vi "shift Scan Pattern.vi"(4 "error in (no error)":errorcluster, 5 "Shift Y":dbl, 6 "Shift X":dbl, 7 "Scan Pattern in":refnum<class "Scan Pattern.lvclass">) -> (0 "error out":errorcluster, 3 "Scan Pattern out":refnum<class "Scan Pattern.lvclass">)   [LabVIEW 2018]
uses:
  SpectralRadar/LabVIEW/2012/user.lib/SpectralRadar.llb/Scan Pattern.lvclass
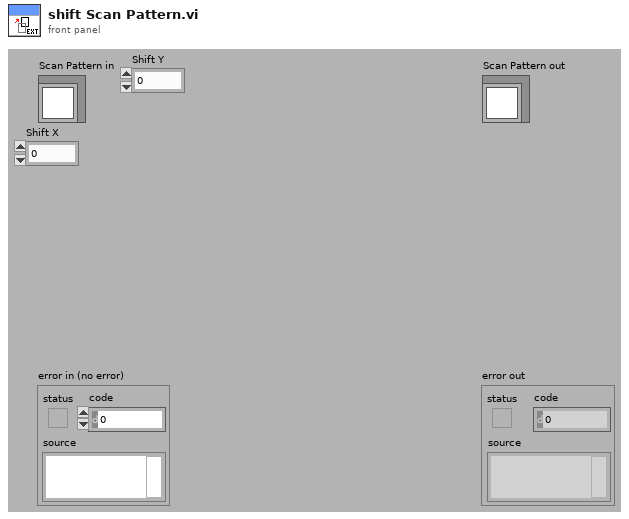
[diagram p1: front panel]
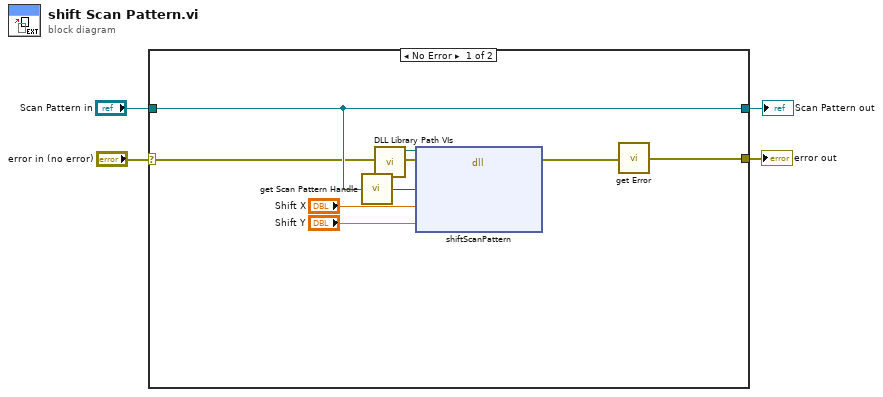
[diagram p0: block diagram]
diagram:
  n1 = case shown="No Error" "error in (no error)" {
    selector: "error in (no error)" -> [w11 w14]
    tunnel: [w6 w14] -> w3
    tunnel: [w12 w13] -> w1
    tunnel: "Scan Pattern in" -> [w12 w13]
    frame No Error {
      n2 = call "get Scan Pattern Handle.vi"("Scan Pattern"=w12) -> ("Handle"=w10:u64)
      n3 = call "DLL Library Path VIs.vi"() -> ("SpectralRadarDLL"=w5:path)  [unwired: 8 in, 3 out]
      n4 = dll-call lib="C:/Project/SerialSectOCT - FFT GPU/SerialSectOCT/Labview Software/DLL/SpectralRadar.dll" fn="shiftScanPattern"(path in=w5, error in=w11, "Scan Pattern Handle"=w10, "Shift X"="Shift X", "Shift Y"="Shift Y") -> (error out=w7:errorcluster)  [unwired: 5 in, 1 out]
      n5 = call "get Error.vi"("error in (no error)"=w7) -> ("error out"=w6:errorcluster)
    }
    frame Error {
    }
  }
  "error out" <- w3
  "Scan Pattern out" <- w1
